vi "EventStructure.vi"() -> ()   [LabVIEW 2012]
panel:
  out "Stop":i32
  in  "Stop Button":bool
  out "Timeout":i32
  out "Count":i32
  in  "Count Button":bool
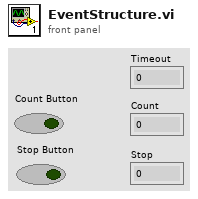
[diagram p1: front panel]
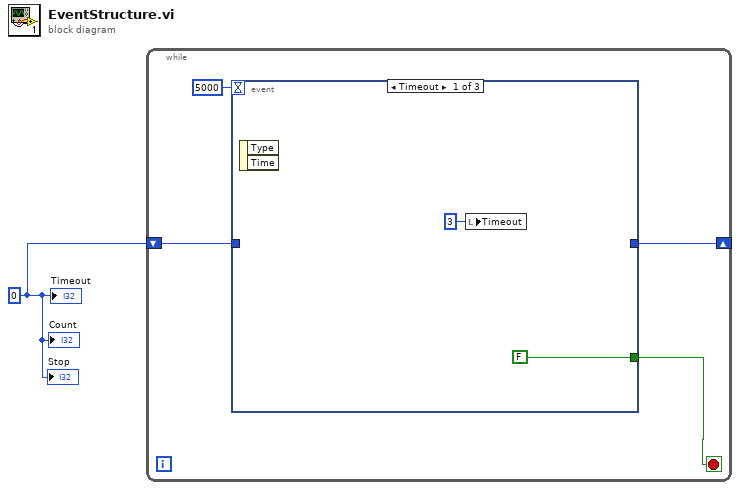
[diagram p0: block diagram]
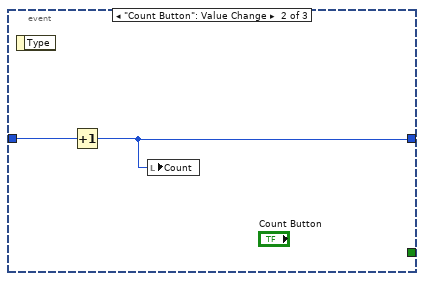
[diagram p2: hidden frame]
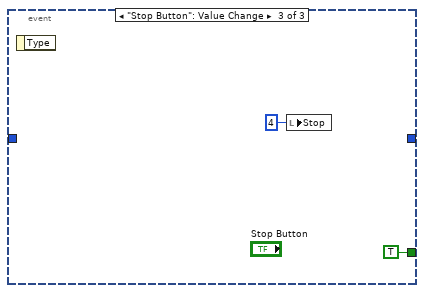
[diagram p3: hidden frame]
diagram:
  w1 = 0 ("Timeout")
  n1 = while {
    shift-right: [w2] -> _
    shift-left: w1 -> [w3]
    stop <- w4 stop-if-true
    n2 = event shown="[0] Timeout" {
      selector: _ -> [_ _ _]
      dyn-events: _ -> [_ _ _]
      timeout: 5000 -> [_ _ _]
      tunnel: [FALSE _ TRUE] -> w4
      tunnel: w3 -> [_ w9 _]
      tunnel: [_ w8 _] -> w2
      event Timeout {
        n3 = event-data() -> ()  [unwired: 1 in, 2 out]
        n4 = local write "Timeout"(3 ("Timeout")) -> ()
      }
      event "Count Button": Value Change {
        n5 = event-data() -> ()  [unwired: 1 in, 1 out]
        n6 = Increment(x=w9) -> (x+1=w8:i32)
        n7 = local write "Count"(w8) -> ()
      }
      event "Stop Button": Value Change {
        n8 = event-data() -> ()  [unwired: 1 in, 1 out]
        n9 = local write "Stop"(4 ("Stop")) -> ()
      }
    }
  }
  "Count" <- w1
  "Timeout" <- w1
  "Stop" <- w1
